vi "Synchronize.vi"(8 "error in (no error)":errorcluster, 10 "Frequency Control":refnum<class "Message Enqueuer.lvclass">, 11 "IED in":refnum<class "IED.lvclass">) -> (0 "error out":errorcluster, 3 "IED out":refnum<class "IED.lvclass">)   [LabVIEW 2015, in "IED Actor.lvlib" / "IED.lvclass"]
uses:
  IED.lvclass
  <vilib>/ActorFramework/Message Enqueuer/Message Enqueuer.lvclass
  Synchronization Actor/Synchronization/Synchronization.lvclass
  <vilib>/ActorFramework/Actor/Actor.lvclass/Actor.ctl
  IED.lvclass/IED.ctl
  Synchronization Actor/Synchronization/Synchronization.lvclass/Synchronization.ctl
  Synchronization Actor/Synchronization/Configuration/Write Activation Start.vi
  Synchronization Actor/Synchronization/Configuration/Write Activation Status.vi
  Synchronization Actor/Synchronization/Configuration/Write Modbus Handle.vi
  Synchronization Actor/Synchronization/Configuration/Write Timeout.vi
  Synchronization Actor/Synchronization/Configuration/Write SCADA Core.vi
  Synchronization Actor/Synchronization/Configuration/Write Frequency Control.vi
  <vilib>/ActorFramework/Actor/Actor.lvclass
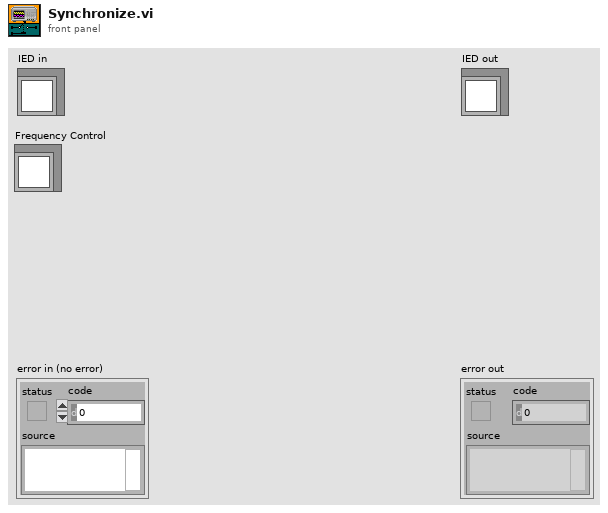
[diagram p1: front panel]
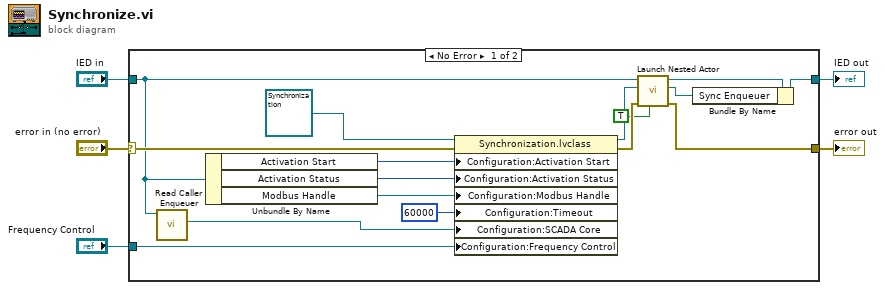
[diagram p0: block diagram]
diagram:
  n1 = case shown="No Error" "error in (no error)" {
    selector: "error in (no error)" -> [w17 w23]
    tunnel: [w13 w23] -> w4
    tunnel: [w7 w22] -> w5
    tunnel: "IED in" -> [w11 w22]
    tunnel: "Frequency Control" -> [w12 _]
    frame No Error {
      n2 = call <vilib>:"Read Caller Enqueuer.vi"("Actor"=w11) -> ("Caller Enqueuer"=w10:refnum<class "Message Enqueuer.lvclass">)  [unwired: 10 in]
      n3 = Unbundle By Name(w11) -> ("Activation Start"=w20:u16, "Activation Status"=w19:u16, "Modbus Handle"=w18:refnum<class "Modbus Master.lvclass">)
      n4 = property class="Synchronization.lvclass"(reference=refnum<class "Synchronization.lvclass"> refnum ("Synchronization Actor.lvlib:Synchronization.lvclass"), error in=w17, "Configuration:Activation Start"=w20, "Configuration:Activation Status"=w19, "Configuration:Modbus Handle"=w18, "Configuration:Timeout"=u32 60000 ("Timeout"), "Configuration:SCADA Core"=w10, "Configuration:Frequency Control"=w12) -> (reference out=w14:refnum<class "Synchronization.lvclass">, error out=w15:errorcluster)
      n5 = call <vilib>:"Launch Nested Actor.vi"("Open Actor Core front panel? (F)"=TRUE, "error in (no error)"=w15, "Nested Actor"=w14, "Caller Actor in"=w11) -> ("error out"=w13:errorcluster, "Nested Actor's Enqueuer"=w6:refnum<class "Message Enqueuer.lvclass">, "Caller Actor out"=w16:refnum<class "IED.lvclass">)  [unwired: 5 in]
      n6 = Bundle By Name(cluster=w16, "Sync Enqueuer"=w6) -> (w7:refnum<class "IED.lvclass">)
    }
    frame Error {
    }
  }
  "error out" <- w4
  "IED out" <- w5
